vi "Configurator v4.vi"() -> ()   [LabVIEW 2019]
uses:
  Sub-VIs/Globals and Definitions/Config Loader TypeDefs/Watch Circle.ctl
  Sub-VIs/Globals and Definitions/Config Loader TypeDefs/Email Settings.ctl
  Sub-VIs/Globals and Definitions/Config Loader TypeDefs/Summary File.ctl
  Sub-VIs/Globals and Definitions/Config Loader TypeDefs/File Settings.ctl
  Sub-VIs/Globals and Definitions/Enum_FileNewInterval.ctl
  Sub-VIs/Globals and Definitions/Config Loader TypeDefs/Watchdog.ctl
  Sub-VIs/Globals and Definitions/Config Loader TypeDefs/AWS and FTP.ctl
  Sub-VIs/Globals and Definitions/TDMS Constants.ctl
  Sub-VIs/Globals and Definitions/Config Loader TypeDefs/All Tab Controls RDv1.0.ctl
  Sub-VIs/Globals and Definitions/Config Loader TypeDefs/Tab Ring.ctl
  <vilib>/Utility/xml.llb/Write to XML File(string).vi
  <vilib>/Utility/xml.llb/Read From XML File(string).vi
panel:
  in  "Tab 7":bool
  in  "Tab 6":bool
  in  "Save":bool=TRUE
  in  "Load":bool=TRUE
  in  "Tab Control":T1(tab)
  in  "Watch Circle":T2={"Set Point Lat (dd)"=39.9132, "Set Point Lon (dd)"=-105.228346, "Yellow Alert Radius (m)"=2.0, "Red Alert Radius (m)"=2.5, "AWOL Radius (m)"=5.0, "Yellow Alert Snooze (min)"=1.0, "Red Alert Snooze (min)"=1.0, "AWOL Radius Snooze (min)"=0.25} {"AWOL Radius Snooze (min)" format="%#_13g"; "Red Alert Snooze (min)" format="%#_13g"; "Yellow Alert Snooze (min)" format="%#_13g"; "AWOL Radius (m)" format="%#_13g"; "Red Alert Radius (m)" format="%#_13g"; "Yellow Alert Radius (m)" format="%#_13g"; "Set Point Lon (dd)" format="%#_13g"; "Set Point Lat (dd)" format="%#_13g"}
  in  "Email Settings":T3
  in  "File Settings":T4={"Config File Path"="/media/sdb1", "Data Folder Path"="/media/sdb1/data", "Raw Mode"="Continuous", "Raw Interval (min)"=10, "Raw Sampling Time (min)"=2, "TDMS File Write Interval"=enum."10 Min", "Default Filename"=path "MODAQ Configuration File.xml", "Enable TDMS Save (3ph only)"=TRUE}
  in  "Summary File":T6={"Enable CSV"=TRUE, "CSV Averaging Time (Sec)"=600, "CSV Loop Delay (ms)"=500}
  in  "FTP and AWS":T7={"AWS Access Key"="", "AWS Secret Key"="", "AWS Bucket"="", "Enable AWS Upload (Summary)"=FALSE, "Enable FTP Upload"=FALSE, "FTP Host"="", "FTP User"="", "FTP Password"="", "Destination write path (pos)"="", "Local file path (pos)"="", "Summary  Upload Interval pos (min)"=10, "Delete Local File After Upload"=FALSE, "Destination write path (pow)"="", "Local file path (pow)"="", "Summary Upload Interval pow (min)"=10, "Enable AWS Upload (TDMS)"=FALSE}
  in  "Watchdog":T8={"Watchdog Period (ms)"=2000, "Reset System on WD timeout"=FALSE, "Enable RT Watchdog"=FALSE}
  in  "Instrument Settings":T9(tab)
  in  "Stbd 3 Phase Current Scaling":dbl[](array[numeric])=[-12.724, -12.739, -12.73]
  in  "Stbd 3 Phase Voltage Scaling":dbl[](array[numeric])=[50.0, 50.0, 50.0]
  in  "PowGrp0 Sampling":T10={"PowGrp0 sample rate [Hz]"=5000.0, "PowGrp0 samples per channel"=2500} {"PowGrp0 sample rate [Hz]" format="%0.2f"}
  in  "Scaling Factors Grp0":dbl[](array[numeric])
  in  "PowGrp0":T11={"Channel Names"=["", "", "", "", "", "", "", "", "", "", "", ""], "Channel Units"=["", "", "", "", "", "", "", "", "", "", "", ""], "TDMS File Suffix"="PowGrp0", "Channel Datatype"=["", "", "", "", "", "", "", "", "", "", "", ""]}
  in  "Quit":bool=TRUE
  in  "Tab 5":bool
  in  "Tab 3":bool=TRUE
  in  "Tab 4":bool=TRUE
  in  "Tab 2":bool
  in  "Tab 1":bool
  # "Watch Circle"
  # "Notifications"
  # "File Preferences"
  # "Upload Destinations"
  # "General Settings"
  # "PT-EN1-1001"
  # "CT-EN1-1001"
  # "PT-EN1-1002"
  # "CT-EN1-1002"
  # "PT-EN1-1003"
  # "CT-EN1-1003"
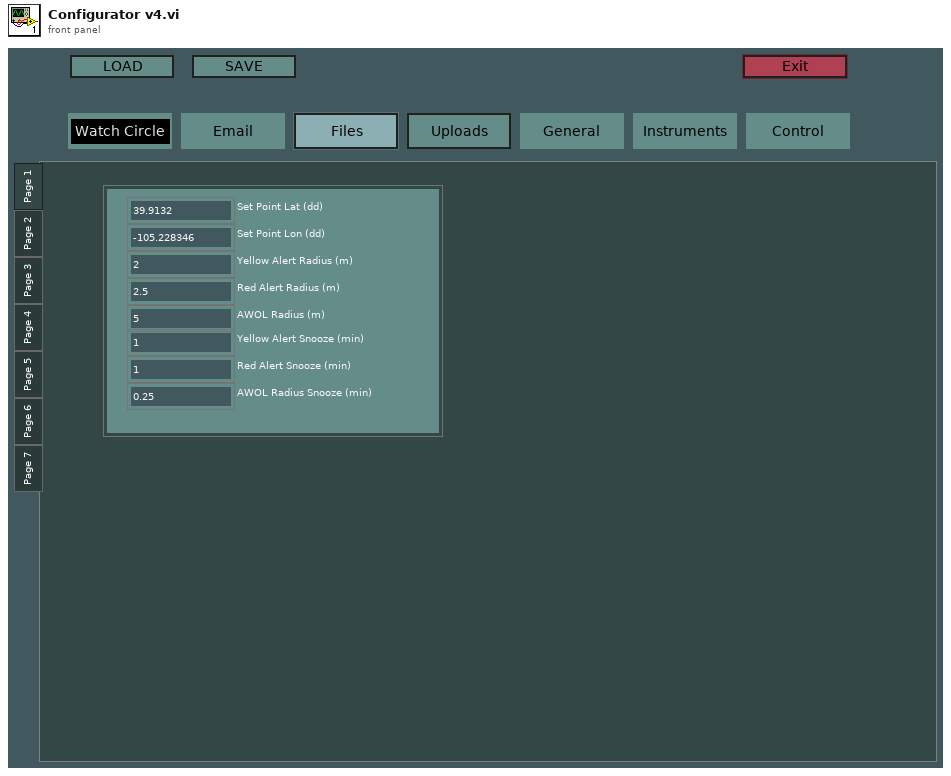
[diagram p1: front panel]
types:
  T1 = enum32{"Page 1", "Page 2", "Page 3", "Page 4", "Page 5", "Page 6", "Page 7"}
  T2 = typedef "Watch Circle.ctl" = cluster{"Set Point Lat (dd)":dbl, "Set Point Lon (dd)":dbl, "Yellow Alert Radius (m)":dbl, "Red Alert Radius (m)":dbl, "AWOL Radius (m)":dbl, "Yellow Alert Snooze (min)":dbl, "Red Alert Snooze (min)":dbl, "AWOL Radius Snooze (min)":dbl}
  T3 = typedef "Email Settings.ctl" = cluster{"Enable Alerts":bool, "Distribution List (comma separated) 1":string, "Distribution List (comma separated) 2":string, "Sender Email":string, "SMTP":string, "Username":string, "Password":string}
  T4 = typedef "File Settings.ctl" = cluster{"Config File Path":string, "Data Folder Path":string, "Raw Mode":string, "Raw Interval (min)":i32, "Raw Sampling Time (min)":i32, "TDMS File Write Interval":T5, "Default Filename":path, "Enable TDMS Save (3ph only)":bool}
  T5 = typedef "Enum_FileNewInterval.ctl" = enum16{"10 Min", "Hourly", "Daily", "Weekly", "Monthly"}
  T6 = typedef "Summary File.ctl" = cluster{"Enable CSV":bool, "CSV Averaging Time (Sec)":i32, "CSV Loop Delay (ms)":i32}
  T7 = typedef "AWS and FTP.ctl" = cluster{"AWS Access Key":string, "AWS Secret Key":string, "AWS Bucket":string, "Enable AWS Upload (Summary)":bool, "Enable FTP Upload":bool, "FTP Host":string, "FTP User":string, "FTP Password":string, "Destination write path (pos)":string, "Local file path (pos)":string, "Summary  Upload Interval pos (min)":i32, "Delete Local File After Upload":bool, "Destination write path (pow)":string, "Local file path (pow)":string, "Summary Upload Interval pow (min)":i32, "Enable AWS Upload (TDMS)":bool}
  T8 = typedef "Watchdog.ctl" = cluster{"Watchdog Period (ms)":u32, "Reset System on WD timeout":bool, "Enable RT Watchdog":bool}
  T9 = enum32{"PTO 1", "PTO 2", "Wave Staff 1", "RTD", "Voltage Inputs", "Encoders", "Loadcells & Strain Gages"}
  T10 = cluster{"PowGrp0 sample rate [Hz]":dbl, "PowGrp0 samples per channel":i32}
  T11 = typedef "TDMS Constants.ctl" = cluster{"Channel Names":string[], "Channel Units":string[], "TDMS File Suffix":string, "Channel Datatype":string[]}
  T12 = typedef "All Tab Controls RDv1.0.ctl" = cluster{"Watch Circle":T2, "FTP and AWS":T7, "Email Settings":T3, "Summary File":T6, "File Settings":T4, "Watchdog":T8, "PowGrp0":T11, "Scaling Factors Grp0":dbl[], "PowGrp0 Sampling":cluster{"PowGrp0 sample rate [Hz]":dbl, "PowGrp0 samples per channel":i32}, "Stbd 3 Phase Voltage Scaling":dbl[], "Stbd 3 Phase Current Scaling":dbl[]}
  T13 = typedef "Tab Ring.ctl" = enum32{"Page 1", "Page 2", "Page 3", "Page 4", "Page 5", "Page 6", "Page 7"}
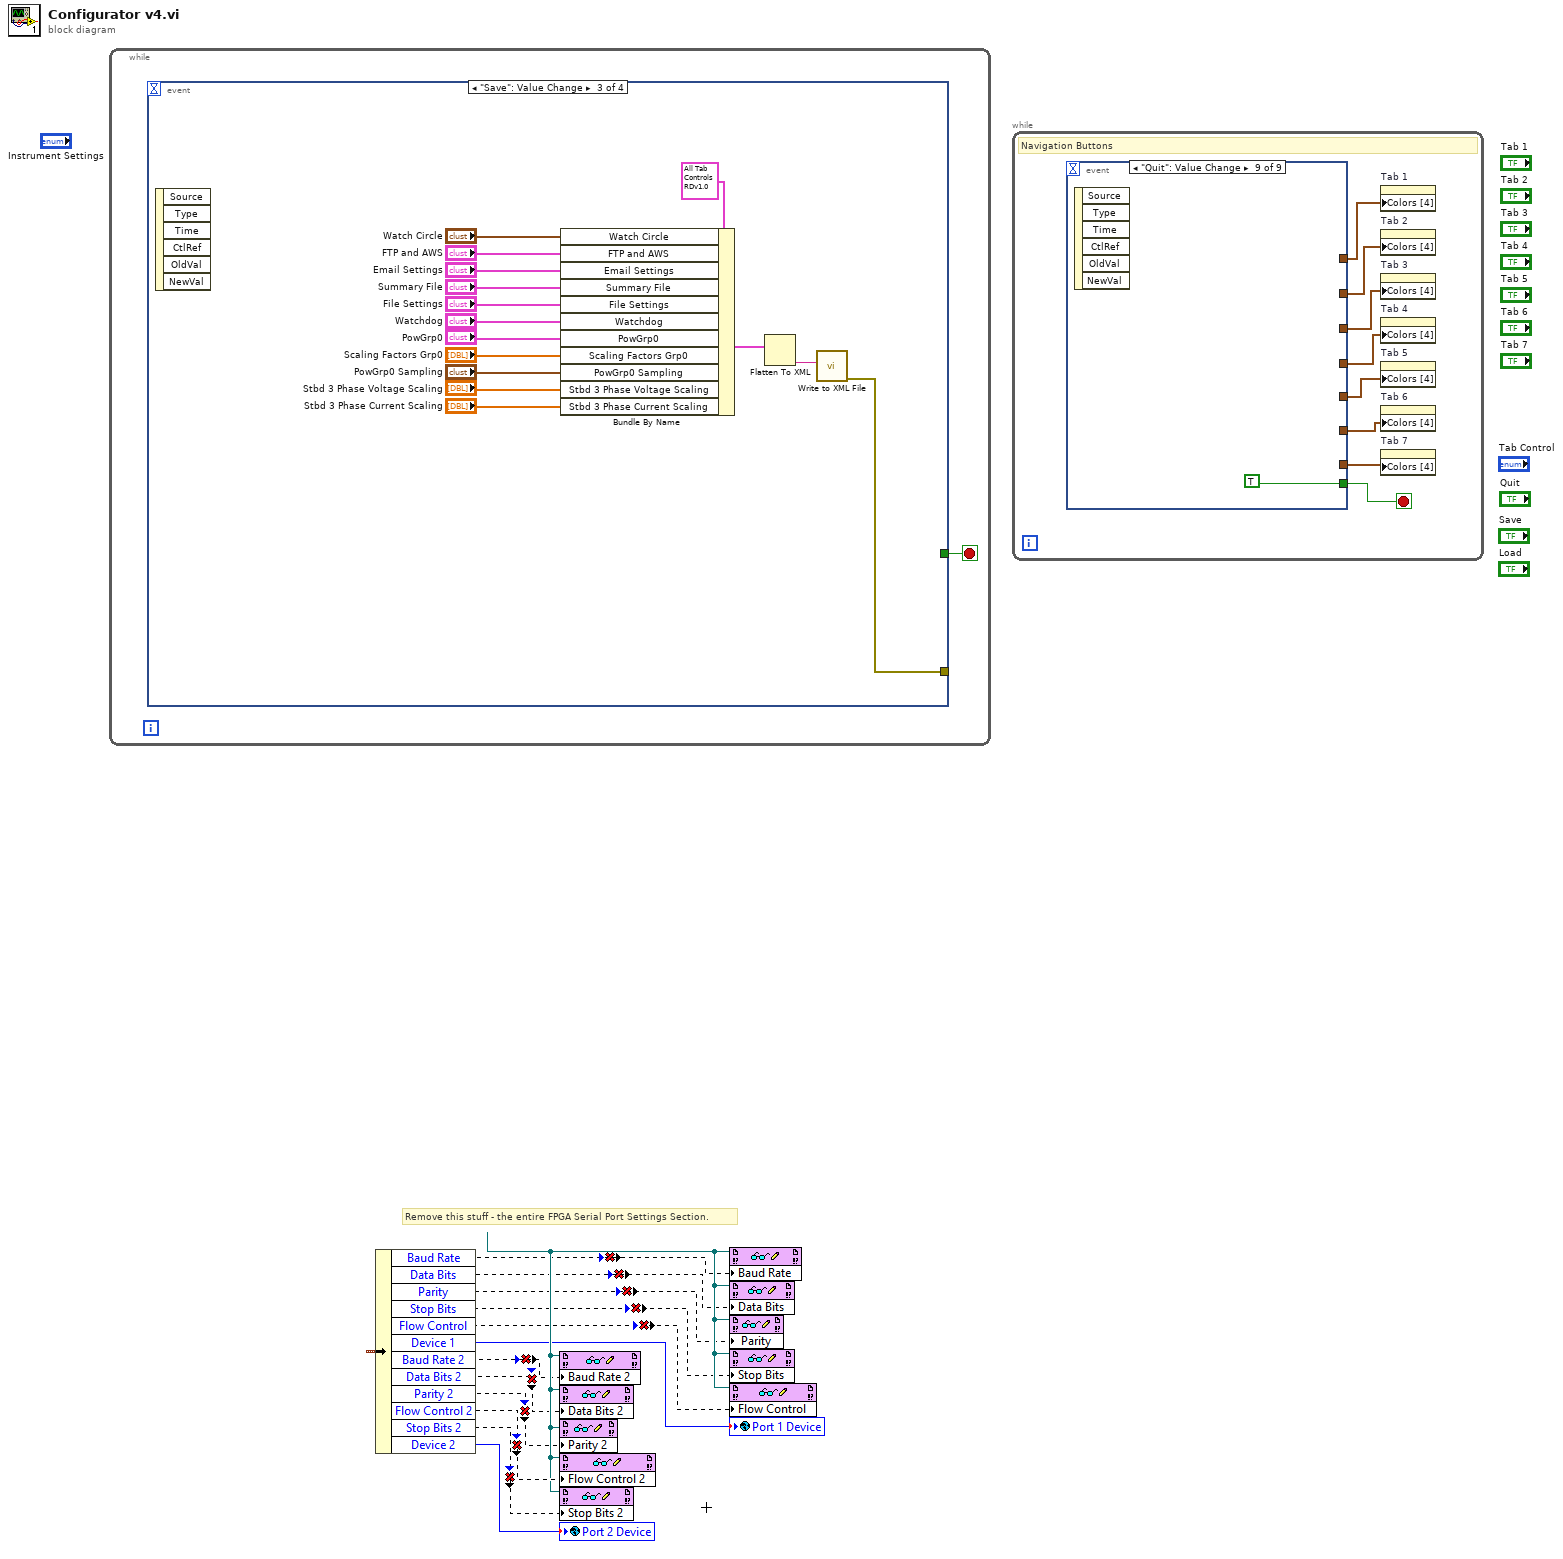
[diagram p0: block diagram]
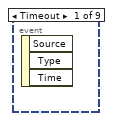
[diagram p2: hidden frame]
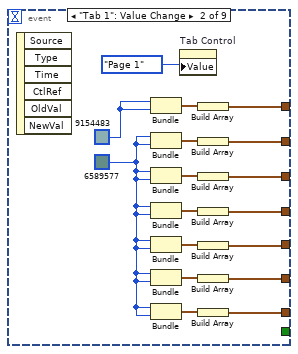
[diagram p3: hidden frame]
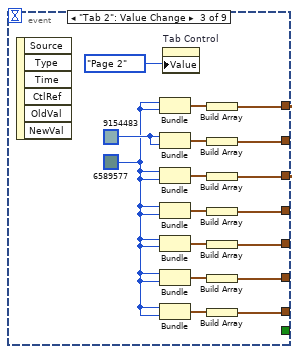
[diagram p4: hidden frame]
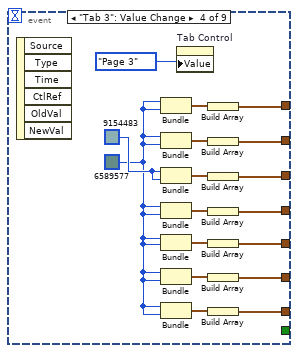
[diagram p5: hidden frame]
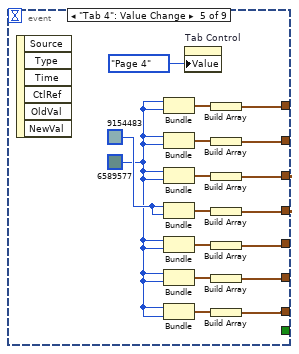
[diagram p6: hidden frame]
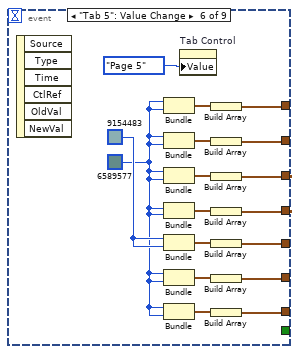
[diagram p7: hidden frame]
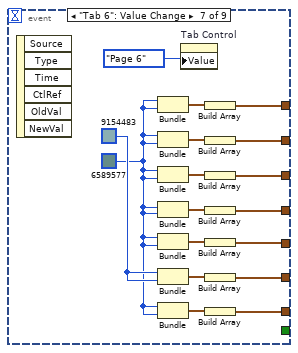
[diagram p8: hidden frame]
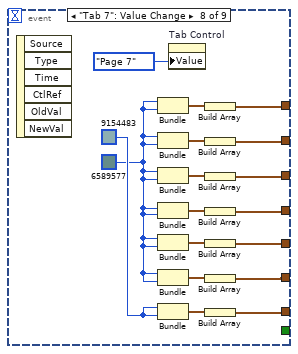
[diagram p9: hidden frame]
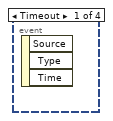
[diagram p10: hidden frame]
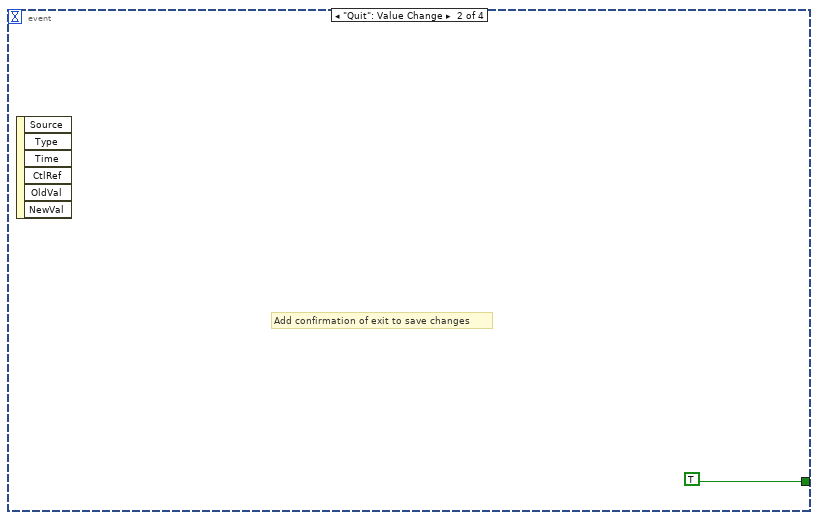
[diagram p11: hidden frame]
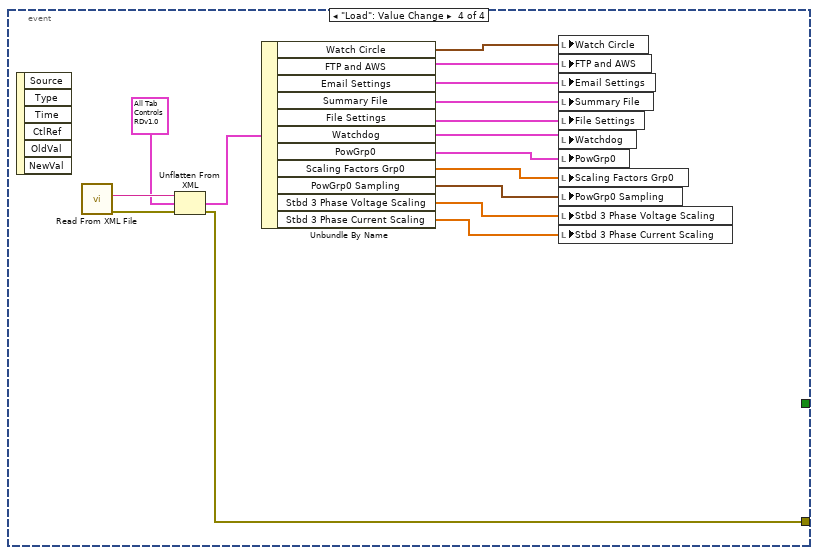
[diagram p12: hidden frame]
diagram:
  # "Remove this stuff - the entire FPGA Serial Port Settings Section."
  n1 = while {
    stop <- w1 stop-if-true
    n2 = event shown="[2] \"Save\": Value Change" {
      selector: _ -> [_ _ _ _]
      dyn-events: _ -> [_ _ _ _]
      timeout: _ -> [_ _ _ _]
      tunnel: [_ TRUE _ _] -> w1
      tunnel: [_ _ w17 w30] -> _
      event Timeout {
        n3 = event-data() -> ()  [unwired: 1 in, 3 out]
      }
      event "Quit": Value Change {
        # "Add confirmation of exit to save changes"
        n4 = event-data() -> ()  [unwired: 1 in, 6 out]
      }
      event "Save": Value Change {
        n5 = event-data() -> ()  [unwired: 1 in, 6 out]
        n6 = Bundle By Name(cluster=T12 {"Watch Circle"={"Set Point Lat (dd)"=0.0, "Set Point Lon (dd)"=0.0, "Yellow Alert Radius (m)"=0.0, "Red Alert Radius (m)"=0.0, "AWOL Radius (m)"=0.0, "Yellow Alert Snooze (min)"=0.0, "Red Alert Snooze (min)"=0.0, "AWOL Radius Snooze (min)"=0.0}, "FTP and AWS"={"AWS Access Key"="", "AWS Secret Key"="", "AWS Bucket"="", "Enable AWS Upload (Summary)"=FALSE, "Enable FTP Upload"=FALSE, "FTP Host"="", "FTP User"="", "FTP Password"="", "Destination write path (pos)"="", "Local file path (pos)"="", "Summary  Upload Interval pos (min)"=0, "Delete Local File After Upload"=FALSE, "Destination write path (pow)"="", "Local file path (pow)"="", "Summary Upload Interval pow (min)"=0, "Enable AWS Upload (TDMS)"=FALSE}, "Email Settings"={"Enable Alerts"=FALSE, "Distribution List (comma separated) 1"="", "Distribution List (comma separated) 2"="", "Sender Email"="", "SMTP"="", "Username"="", "Password"=""}, "Summary File"={"Enable CSV"=FALSE, "CSV Averaging Time (Sec)"=0, "CSV Loop Delay (ms)"=0}, "File Settings"={"Config File Path"="", "Data Folder Path"="", "Raw Mode"="", "Raw Interval (min)"=0, "Raw Sampling Time (min)"=0, "TDMS File Write Interval"=enum."10 Min", "Default Filename"=path "MODAQ Configuration File.ini", "Enable TDMS Save (3ph only)"=FALSE}, "Watchdog"={"Watchdog Period (ms)"=1000, "Reset System on WD timeout"=FALSE, "Enable RT Watchdog"=FALSE}, "PowGrp0"={"Channel Names"=["CT-EN6-2003", "CT-EN6-3001", "CT-EN6-3002", "PT-EN6-1001", "CT-EN1-1005", "CT-EN2-1005", "CT-EN6-2001", "CT-EN6-2002", "PT-EN6-1002", "CT-EN7-1001", "PT-EN7-1001", "TimeStamp"], "Channel Units"=["ADC", "ADC", "ADC", "VDC", "ADC", "ADC", "ADC", "ADC", "VDC", "ADC", "VDC", "UTC"], "TDMS File Suffix"="PowGrp2", "Channel Datatype"=["Float", "Float", "Float", "Float", "Float", "Float", "Float", "Float", "Float", "Float", "Float", "Float"]}, "Scaling Factors Grp0"=[], "PowGrp0 Sampling"={"PowGrp0 sample rate [Hz]"=5000.0, "PowGrp0 samples per channel"=500}, "Stbd 3 Phase Voltage Scaling"=[50.0, 50.0, 50.0], "Stbd 3 Phase Current Scaling"=[-12.724, -12.739, -12.73]} ("All Controls"), "Watch Circle"="Watch Circle", "FTP and AWS"="FTP and AWS", "Email Settings"="Email Settings", "Summary File"="Summary File", "File Settings"="File Settings", "Watchdog"="Watchdog", "PowGrp0"="PowGrp0", "Scaling Factors Grp0"="Scaling Factors Grp0", "PowGrp0 Sampling"="PowGrp0 Sampling", "Stbd 3 Phase Voltage Scaling"="Stbd 3 Phase Voltage Scaling", "Stbd 3 Phase Current Scaling"="Stbd 3 Phase Current Scaling") -> (w15:T12)
        n7 = Flatten To XML(anything=w15) -> (xml string=w16:string)
        n8 = call-poly <vilib>:"Write to XML File.vi"("XML Input"=w16) -> ("error out"=w17:errorcluster)  [unwired: 8 in, 2 out]
      }
      event "Load": Value Change {
        n9 = event-data() -> ()  [unwired: 1 in, 6 out]
        n10 = call-poly <vilib>:"Read From XML File.vi"() -> ("error out"=w31:errorcluster, "XML Elements"=w33:string)  [unwired: 9 in, 1 out]
        n11 = Unflatten From XML(xml string=w33, type=T12 {"Watch Circle"={"Set Point Lat (dd)"=0.0, "Set Point Lon (dd)"=0.0, "Yellow Alert Radius (m)"=0.0, "Red Alert Radius (m)"=0.0, "AWOL Radius (m)"=0.0, "Yellow Alert Snooze (min)"=0.0, "Red Alert Snooze (min)"=0.0, "AWOL Radius Snooze (min)"=0.0}, "FTP and AWS"={"AWS Access Key"="", "AWS Secret Key"="", "AWS Bucket"="", "Enable AWS Upload (Summary)"=FALSE, "Enable FTP Upload"=FALSE, "FTP Host"="", "FTP User"="", "FTP Password"="", "Destination write path (pos)"="", "Local file path (pos)"="", "Summary  Upload Interval pos (min)"=0, "Delete Local File After Upload"=FALSE, "Destination write path (pow)"="", "Local file path (pow)"="", "Summary Upload Interval pow (min)"=0, "Enable AWS Upload (TDMS)"=FALSE}, "Email Settings"={"Enable Alerts"=FALSE, "Distribution List (comma separated) 1"="", "Distribution List (comma separated) 2"="", "Sender Email"="", "SMTP"="", "Username"="", "Password"=""}, "Summary File"={"Enable CSV"=FALSE, "CSV Averaging Time (Sec)"=0, "CSV Loop Delay (ms)"=0}, "File Settings"={"Config File Path"="", "Data Folder Path"="", "Raw Mode"="", "Raw Interval (min)"=0, "Raw Sampling Time (min)"=0, "TDMS File Write Interval"=enum."10 Min", "Default Filename"=path "MODAQ Configuration File.ini", "Enable TDMS Save (3ph only)"=FALSE}, "Watchdog"={"Watchdog Period (ms)"=1000, "Reset System on WD timeout"=FALSE, "Enable RT Watchdog"=FALSE}, "PowGrp0"={"Channel Names"=["CT-EN6-2003", "CT-EN6-3001", "CT-EN6-3002", "PT-EN6-1001", "CT-EN1-1005", "CT-EN2-1005", "CT-EN6-2001", "CT-EN6-2002", "PT-EN6-1002", "CT-EN7-1001", "PT-EN7-1001", "TimeStamp"], "Channel Units"=["ADC", "ADC", "ADC", "VDC", "ADC", "ADC", "ADC", "ADC", "VDC", "ADC", "VDC", "UTC"], "TDMS File Suffix"="PowGrp2", "Channel Datatype"=["Float", "Float", "Float", "Float", "Float", "Float", "Float", "Float", "Float", "Float", "Float", "Float"]}, "Scaling Factors Grp0"=[], "PowGrp0 Sampling"={"PowGrp0 sample rate [Hz]"=5000.0, "PowGrp0 samples per channel"=500}, "Stbd 3 Phase Voltage Scaling"=[50.0, 50.0, 50.0], "Stbd 3 Phase Current Scaling"=[-12.724, -12.739, -12.73]} ("All Controls"), error in (no error)=w31) -> (value=w32:T12, error out=w30:errorcluster)
        n12 = Unbundle By Name(w32) -> ("Watch Circle"=w29:T2, "FTP and AWS"=w24:T7, "Email Settings"=w28:T3, "Summary File"=w27:T6, "File Settings"=w26:T4, "Watchdog"=w25:T8, "PowGrp0"=w23:T11, "Scaling Factors Grp0"=w22:dbl[], "PowGrp0 Sampling"=w21:T10, "Stbd 3 Phase Voltage Scaling"=w19:dbl[], "Stbd 3 Phase Current Scaling"=w18:dbl[])
        n13 = local write "Watch Circle"(w29) -> ()
        n14 = local write "FTP and AWS"(w24) -> ()
        n15 = local write "Email Settings"(w28) -> ()
        n16 = local write "Summary File"(w27) -> ()
        n17 = local write "File Settings"(w26) -> ()
        n18 = local write "Watchdog"(w25) -> ()
        n19 = local write "PowGrp0"(w23) -> ()
        n20 = local write "Scaling Factors Grp0"(w22) -> ()
        n21 = local write "PowGrp0 Sampling"(w21) -> ()
        n22 = local write "Stbd 3 Phase Voltage Scaling"(w19) -> ()
        n23 = local write "Stbd 3 Phase Current Scaling"(w18) -> ()
      }
    }
  }
  n24 = while {
    stop <- w41 stop-if-true
    # "Navigation Buttons"
    n25 = event shown="[8] \"Quit\": Value Change" {
      selector: _ -> [_ _ _ _ _ _ _ _ _]
      dyn-events: _ -> [_ _ _ _ _ _ _ _ _]
      timeout: _ -> [_ _ _ _ _ _ _ _ _]
      tunnel: [_ _ _ _ _ _ _ _ TRUE] -> w41
      tunnel: [_ w53 w71 w88 w105 w122 w136 w153 _] -> w37
      tunnel: [_ w52 w70 w87 w104 w121 w135 w152 _] -> w38
      tunnel: [_ w51 w69 w86 w103 w120 w134 w151 _] -> w40
      tunnel: [_ w50 w68 w85 w102 w119 w133 w150 _] -> w39
      tunnel: [_ w48 w65 w82 w99 w117 w132 w149 _] -> w36
      tunnel: [_ w44 w61 w78 w95 w112 w131 w148 _] -> w35
      tunnel: [_ w43 w60 w77 w94 w111 w130 w147 _] -> w34
      event Timeout {
        n26 = event-data() -> ()  [unwired: 1 in, 3 out]
      }
      event "Tab 1": Value Change {
        w54 = u32 9154483 ("Color Box")
        w45 = u32 6589577 ("Color Box")
        n27 = event-data() -> ()  [unwired: 1 in, 6 out]
        n28 = Bundle("Color Box"=w54, "Color Box"=w54) -> (w58:cluster{"Color Box":u32, "Color Box":u32})  [unwired: 1 in]
        n29 = Bundle("Color Box"=w45, "Color Box"=w45) -> (w57:cluster{"Color Box":u32, "Color Box":u32})  [unwired: 1 in]
        n30 = Bundle("Color Box"=w45, "Color Box"=w45) -> (w56:cluster{"Color Box":u32, "Color Box":u32})  [unwired: 1 in]
        n31 = Bundle("Color Box"=w45, "Color Box"=w45) -> (w55:cluster{"Color Box":u32, "Color Box":u32})  [unwired: 1 in]
        n32 = Bundle("Color Box"=w45, "Color Box"=w45) -> (w49:cluster{"Color Box":u32, "Color Box":u32})  [unwired: 1 in]
        n33 = Bundle("Color Box"=w45, "Color Box"=w45) -> (w47:cluster{"Color Box":u32, "Color Box":u32})  [unwired: 1 in]
        n34 = Bundle("Color Box"=w45, "Color Box"=w45) -> (w46:cluster{"Color Box":u32, "Color Box":u32})  [unwired: 1 in]
        n35 = property on="Tab Control" class="TabCtl (strict)"("Value"=Tab_Ring."Page 1" ("Tab Control")) -> ()  [unwired: 2 in, 2 out]
        n36 = Build Array(w58) -> (w53:cluster{"Color Box":u32, "Color Box":u32}[])
        n37 = Build Array(w57) -> (w52:cluster{"Color Box":u32, "Color Box":u32}[])
        n38 = Build Array(w56) -> (w51:cluster{"Color Box":u32, "Color Box":u32}[])
        n39 = Build Array(w55) -> (w50:cluster{"Color Box":u32, "Color Box":u32}[])
        n40 = Build Array(w49) -> (w48:cluster{"Color Box":u32, "Color Box":u32}[])
        n41 = Build Array(w47) -> (w44:cluster{"Color Box":u32, "Color Box":u32}[])
        n42 = Build Array(w46) -> (w43:cluster{"Color Box":u32, "Color Box":u32}[])
      }
      event "Tab 2": Value Change {
        w67 = u32 9154483 ("Color Box")
        w62 = u32 6589577 ("Color Box")
        n43 = event-data() -> ()  [unwired: 1 in, 6 out]
        n44 = Bundle("Color Box"=w62, "Color Box"=w62) -> (w75:cluster{"Color Box":u32, "Color Box":u32})  [unwired: 1 in]
        n45 = Bundle("Color Box"=w67, "Color Box"=w67) -> (w74:cluster{"Color Box":u32, "Color Box":u32})  [unwired: 1 in]
        n46 = Bundle("Color Box"=w62, "Color Box"=w62) -> (w73:cluster{"Color Box":u32, "Color Box":u32})  [unwired: 1 in]
        n47 = Bundle("Color Box"=w62, "Color Box"=w62) -> (w72:cluster{"Color Box":u32, "Color Box":u32})  [unwired: 1 in]
        n48 = Bundle("Color Box"=w62, "Color Box"=w62) -> (w66:cluster{"Color Box":u32, "Color Box":u32})  [unwired: 1 in]
        n49 = Bundle("Color Box"=w62, "Color Box"=w62) -> (w64:cluster{"Color Box":u32, "Color Box":u32})  [unwired: 1 in]
        n50 = Bundle("Color Box"=w62, "Color Box"=w62) -> (w63:cluster{"Color Box":u32, "Color Box":u32})  [unwired: 1 in]
        n51 = property on="Tab Control" class="TabCtl (strict)"("Value"=Tab_Ring."Page 2" ("Tab Control")) -> ()  [unwired: 2 in, 2 out]
        n52 = Build Array(w75) -> (w71:cluster{"Color Box":u32, "Color Box":u32}[])
        n53 = Build Array(w74) -> (w70:cluster{"Color Box":u32, "Color Box":u32}[])
        n54 = Build Array(w73) -> (w69:cluster{"Color Box":u32, "Color Box":u32}[])
        n55 = Build Array(w72) -> (w68:cluster{"Color Box":u32, "Color Box":u32}[])
        n56 = Build Array(w66) -> (w65:cluster{"Color Box":u32, "Color Box":u32}[])
        n57 = Build Array(w64) -> (w61:cluster{"Color Box":u32, "Color Box":u32}[])
        n58 = Build Array(w63) -> (w60:cluster{"Color Box":u32, "Color Box":u32}[])
      }
      event "Tab 3": Value Change {
        w84 = u32 9154483 ("Color Box")
        w79 = u32 6589577 ("Color Box")
        n59 = event-data() -> ()  [unwired: 1 in, 6 out]
        n60 = Bundle("Color Box"=w79, "Color Box"=w79) -> (w92:cluster{"Color Box":u32, "Color Box":u32})  [unwired: 1 in]
        n61 = Bundle("Color Box"=w79, "Color Box"=w79) -> (w91:cluster{"Color Box":u32, "Color Box":u32})  [unwired: 1 in]
        n62 = Bundle("Color Box"=w84, "Color Box"=w84) -> (w90:cluster{"Color Box":u32, "Color Box":u32})  [unwired: 1 in]
        n63 = Bundle("Color Box"=w79, "Color Box"=w79) -> (w89:cluster{"Color Box":u32, "Color Box":u32})  [unwired: 1 in]
        n64 = Bundle("Color Box"=w79, "Color Box"=w79) -> (w83:cluster{"Color Box":u32, "Color Box":u32})  [unwired: 1 in]
        n65 = Bundle("Color Box"=w79, "Color Box"=w79) -> (w81:cluster{"Color Box":u32, "Color Box":u32})  [unwired: 1 in]
        n66 = Bundle("Color Box"=w79, "Color Box"=w79) -> (w80:cluster{"Color Box":u32, "Color Box":u32})  [unwired: 1 in]
        n67 = property on="Tab Control" class="TabCtl (strict)"("Value"=Tab_Ring."Page 3" ("Tab Control")) -> ()  [unwired: 2 in, 2 out]
        n68 = Build Array(w92) -> (w88:cluster{"Color Box":u32, "Color Box":u32}[])
        n69 = Build Array(w91) -> (w87:cluster{"Color Box":u32, "Color Box":u32}[])
        n70 = Build Array(w90) -> (w86:cluster{"Color Box":u32, "Color Box":u32}[])
        n71 = Build Array(w89) -> (w85:cluster{"Color Box":u32, "Color Box":u32}[])
        n72 = Build Array(w83) -> (w82:cluster{"Color Box":u32, "Color Box":u32}[])
        n73 = Build Array(w81) -> (w78:cluster{"Color Box":u32, "Color Box":u32}[])
        n74 = Build Array(w80) -> (w77:cluster{"Color Box":u32, "Color Box":u32}[])
      }
      event "Tab 4": Value Change {
        w101 = u32 9154483 ("Color Box")
        w96 = u32 6589577 ("Color Box")
        n75 = event-data() -> ()  [unwired: 1 in, 6 out]
        n76 = Bundle("Color Box"=w96, "Color Box"=w96) -> (w109:cluster{"Color Box":u32, "Color Box":u32})  [unwired: 1 in]
        n77 = Bundle("Color Box"=w96, "Color Box"=w96) -> (w108:cluster{"Color Box":u32, "Color Box":u32})  [unwired: 1 in]
        n78 = Bundle("Color Box"=w96, "Color Box"=w96) -> (w107:cluster{"Color Box":u32, "Color Box":u32})  [unwired: 1 in]
        n79 = Bundle("Color Box"=w101, "Color Box"=w101) -> (w106:cluster{"Color Box":u32, "Color Box":u32})  [unwired: 1 in]
        n80 = Bundle("Color Box"=w96, "Color Box"=w96) -> (w100:cluster{"Color Box":u32, "Color Box":u32})  [unwired: 1 in]
        n81 = Bundle("Color Box"=w96, "Color Box"=w96) -> (w98:cluster{"Color Box":u32, "Color Box":u32})  [unwired: 1 in]
        n82 = Bundle("Color Box"=w96, "Color Box"=w96) -> (w97:cluster{"Color Box":u32, "Color Box":u32})  [unwired: 1 in]
        n83 = property on="Tab Control" class="TabCtl (strict)"("Value"=Tab_Ring."Page 4" ("Tab Control")) -> ()  [unwired: 2 in, 2 out]
        n84 = Build Array(w109) -> (w105:cluster{"Color Box":u32, "Color Box":u32}[])
        n85 = Build Array(w108) -> (w104:cluster{"Color Box":u32, "Color Box":u32}[])
        n86 = Build Array(w107) -> (w103:cluster{"Color Box":u32, "Color Box":u32}[])
        n87 = Build Array(w106) -> (w102:cluster{"Color Box":u32, "Color Box":u32}[])
        n88 = Build Array(w100) -> (w99:cluster{"Color Box":u32, "Color Box":u32}[])
        n89 = Build Array(w98) -> (w95:cluster{"Color Box":u32, "Color Box":u32}[])
        n90 = Build Array(w97) -> (w94:cluster{"Color Box":u32, "Color Box":u32}[])
      }
      event "Tab 5": Value Change {
        w116 = u32 9154483 ("Color Box")
        w113 = u32 6589577 ("Color Box")
        n91 = event-data() -> ()  [unwired: 1 in, 6 out]
        n92 = Bundle("Color Box"=w113, "Color Box"=w113) -> (w126:cluster{"Color Box":u32, "Color Box":u32})  [unwired: 1 in]
        n93 = Bundle("Color Box"=w113, "Color Box"=w113) -> (w125:cluster{"Color Box":u32, "Color Box":u32})  [unwired: 1 in]
        n94 = Bundle("Color Box"=w113, "Color Box"=w113) -> (w124:cluster{"Color Box":u32, "Color Box":u32})  [unwired: 1 in]
        n95 = Bundle("Color Box"=w113, "Color Box"=w113) -> (w123:cluster{"Color Box":u32, "Color Box":u32})  [unwired: 1 in]
        n96 = Bundle("Color Box"=w116, "Color Box"=w116) -> (w118:cluster{"Color Box":u32, "Color Box":u32})  [unwired: 1 in]
        n97 = Bundle("Color Box"=w113, "Color Box"=w113) -> (w115:cluster{"Color Box":u32, "Color Box":u32})  [unwired: 1 in]
        n98 = Bundle("Color Box"=w113, "Color Box"=w113) -> (w114:cluster{"Color Box":u32, "Color Box":u32})  [unwired: 1 in]
        n99 = property on="Tab Control" class="TabCtl (strict)"("Value"=Tab_Ring."Page 5" ("Tab Control")) -> ()  [unwired: 2 in, 2 out]
        n100 = Build Array(w126) -> (w122:cluster{"Color Box":u32, "Color Box":u32}[])
        n101 = Build Array(w125) -> (w121:cluster{"Color Box":u32, "Color Box":u32}[])
        n102 = Build Array(w124) -> (w120:cluster{"Color Box":u32, "Color Box":u32}[])
        n103 = Build Array(w123) -> (w119:cluster{"Color Box":u32, "Color Box":u32}[])
        n104 = Build Array(w118) -> (w117:cluster{"Color Box":u32, "Color Box":u32}[])
        n105 = Build Array(w115) -> (w112:cluster{"Color Box":u32, "Color Box":u32}[])
        n106 = Build Array(w114) -> (w111:cluster{"Color Box":u32, "Color Box":u32}[])
      }
      event "Tab 6": Value Change {
        w129 = u32 9154483 ("Color Box")
        w128 = u32 6589577 ("Color Box")
        n107 = event-data() -> ()  [unwired: 1 in, 6 out]
        n108 = Bundle("Color Box"=w128, "Color Box"=w128) -> (w143:cluster{"Color Box":u32, "Color Box":u32})  [unwired: 1 in]
        n109 = Bundle("Color Box"=w128, "Color Box"=w128) -> (w142:cluster{"Color Box":u32, "Color Box":u32})  [unwired: 1 in]
        n110 = Bundle("Color Box"=w128, "Color Box"=w128) -> (w141:cluster{"Color Box":u32, "Color Box":u32})  [unwired: 1 in]
        n111 = Bundle("Color Box"=w128, "Color Box"=w128) -> (w140:cluster{"Color Box":u32, "Color Box":u32})  [unwired: 1 in]
        n112 = Bundle("Color Box"=w128, "Color Box"=w128) -> (w139:cluster{"Color Box":u32, "Color Box":u32})  [unwired: 1 in]
        n113 = Bundle("Color Box"=w129, "Color Box"=w129) -> (w138:cluster{"Color Box":u32, "Color Box":u32})  [unwired: 1 in]
        n114 = Bundle("Color Box"=w128, "Color Box"=w128) -> (w137:cluster{"Color Box":u32, "Color Box":u32})  [unwired: 1 in]
        n115 = property on="Tab Control" class="TabCtl (strict)"("Value"=Tab_Ring."Page 6" ("Tab Control")) -> ()  [unwired: 2 in, 2 out]
        n116 = Build Array(w143) -> (w136:cluster{"Color Box":u32, "Color Box":u32}[])
        n117 = Build Array(w142) -> (w135:cluster{"Color Box":u32, "Color Box":u32}[])
        n118 = Build Array(w141) -> (w134:cluster{"Color Box":u32, "Color Box":u32}[])
        n119 = Build Array(w140) -> (w133:cluster{"Color Box":u32, "Color Box":u32}[])
        n120 = Build Array(w139) -> (w132:cluster{"Color Box":u32, "Color Box":u32}[])
        n121 = Build Array(w138) -> (w131:cluster{"Color Box":u32, "Color Box":u32}[])
        n122 = Build Array(w137) -> (w130:cluster{"Color Box":u32, "Color Box":u32}[])
      }
      event "Tab 7": Value Change {
        w146 = u32 9154483 ("Color Box")
        w145 = u32 6589577 ("Color Box")
        n123 = event-data() -> ()  [unwired: 1 in, 6 out]
        n124 = Bundle("Color Box"=w145, "Color Box"=w145) -> (w160:cluster{"Color Box":u32, "Color Box":u32})  [unwired: 1 in]
        n125 = Bundle("Color Box"=w145, "Color Box"=w145) -> (w159:cluster{"Color Box":u32, "Color Box":u32})  [unwired: 1 in]
        n126 = Bundle("Color Box"=w145, "Color Box"=w145) -> (w158:cluster{"Color Box":u32, "Color Box":u32})  [unwired: 1 in]
        n127 = Bundle("Color Box"=w145, "Color Box"=w145) -> (w157:cluster{"Color Box":u32, "Color Box":u32})  [unwired: 1 in]
        n128 = Bundle("Color Box"=w145, "Color Box"=w145) -> (w156:cluster{"Color Box":u32, "Color Box":u32})  [unwired: 1 in]
        n129 = Bundle("Color Box"=w145, "Color Box"=w145) -> (w155:cluster{"Color Box":u32, "Color Box":u32})  [unwired: 1 in]
        n130 = Bundle("Color Box"=w146, "Color Box"=w146) -> (w154:cluster{"Color Box":u32, "Color Box":u32})  [unwired: 1 in]
        n131 = property on="Tab Control" class="TabCtl (strict)"("Value"=Tab_Ring."Page 7" ("Tab Control")) -> ()  [unwired: 2 in, 2 out]
        n132 = Build Array(w160) -> (w153:cluster{"Color Box":u32, "Color Box":u32}[])
        n133 = Build Array(w159) -> (w152:cluster{"Color Box":u32, "Color Box":u32}[])
        n134 = Build Array(w158) -> (w151:cluster{"Color Box":u32, "Color Box":u32}[])
        n135 = Build Array(w157) -> (w150:cluster{"Color Box":u32, "Color Box":u32}[])
        n136 = Build Array(w156) -> (w149:cluster{"Color Box":u32, "Color Box":u32}[])
        n137 = Build Array(w155) -> (w148:cluster{"Color Box":u32, "Color Box":u32}[])
        n138 = Build Array(w154) -> (w147:cluster{"Color Box":u32, "Color Box":u32}[])
      }
      event "Quit": Value Change {
        n139 = event-data() -> ()  [unwired: 1 in, 6 out]
      }
    }
    n140 = property on="Tab 1" class="Bool (strict)"("Colors [4]"=w37) -> ()  [unwired: 2 in, 2 out]
    n141 = property on="Tab 2" class="Bool"("Colors [4]"=w38) -> ()  [unwired: 2 in, 2 out]
    n142 = property on="Tab 3" class="Bool"("Colors [4]"=w40) -> ()  [unwired: 2 in, 2 out]
    n143 = property on="Tab 4" class="Bool"("Colors [4]"=w39) -> ()  [unwired: 2 in, 2 out]
    n144 = property on="Tab 5" class="Bool"("Colors [4]"=w36) -> ()  [unwired: 2 in, 2 out]
    n145 = property on="Tab 6" class="Bool"("Colors [4]"=w35) -> ()  [unwired: 2 in, 2 out]
    n146 = property on="Tab 7" class="Bool"("Colors [4]"=w34) -> ()  [unwired: 2 in, 2 out]
  }
